vi "Validate Password.vi"(8 "error in (no error)":errorcluster, 9 "Encoded Password":string, 10 "Plain Password":string, 11 "BasicPasswordEncoder in":refnum<class "BasicPasswordEncoder.lvclass">) -> (0 "error out":errorcluster, 2 "Valid":bool, 3 "BasicPasswordEncoder out":refnum<class "BasicPasswordEncoder.lvclass">)   [LabVIEW 2020, in "HTTP Server.lvlib" / "BasicPasswordEncoder.lvclass"]
uses:
  BasicPasswordEncoder.lvclass
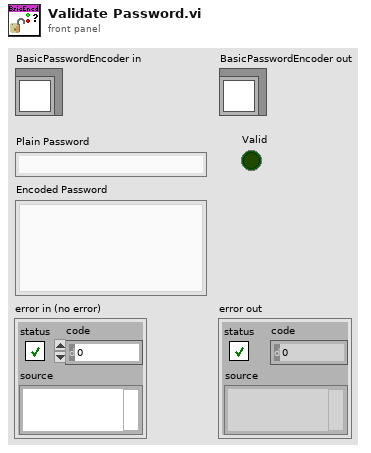
[diagram p1: front panel]
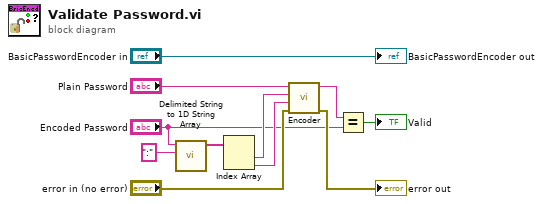
[diagram p0: block diagram]
diagram:
  n1 = call <vilib>:"Delimited String to 1D String Array.vi"("delimiter"=":", "delimited string"="Encoded Password") -> ("string array"=w8:string[])  [unwired: 9 in]
  n2 = Index Array(array=w8) -> (element #1=w7:string, element #2=w6:string)  [unwired: 2 in]
  n3 = call "Encoder.vi"("error in (no error)"="error in (no error)", "Salt 2"=w6, "Salt 1"=w7, "Plain Password"="Plain Password") -> ("error out"=→"error out":errorcluster, "Encoded Password"=w3:string)  [unwired: 6 in]
  n4 = Equal?(x=w3, y="Encoded Password") -> (x = y?=→"Valid":bool)
  "BasicPasswordEncoder out" <- "BasicPasswordEncoder in"
